vi "Convert Time Stamp to String.vi"(10 "time stamp":timestamp format="%<%Y-%m-%dT%H:%M:%S%8u\nTime zone offset %z>T") -> (3 "date/time string":string)   [LabVIEW 2020, in "infolib.lvlib"]
doc: "Converts time stamp into ISO8601 string."
uses:
  infolib.lvlib
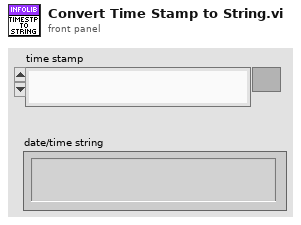
[diagram p1: front panel]
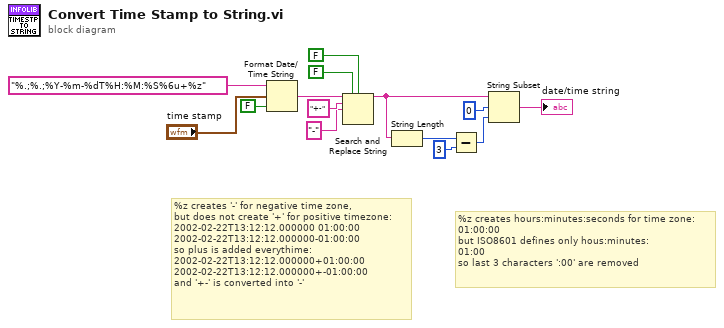
[diagram p0: block diagram]
diagram:
  # "%z creates hours:minutes:seconds for time zone:\n01:00:00\nbut ISO8601 defines only hous:minutes:\n01:00\nso last 3 characters ':00' are removed"
  # "%z creates '-' for negative time zone,\nbut does not create '+' for positive timezone:\n2002-02-22T13:12:12.000000 01:00:00\n2002-02-22T13:12:12.000000-01:00:00\nso plus is added everythime:\n2002-02-22T13:12:12.000000+01:00:00\n2002-02-22T13:12:12.000000+-01:00:00\nand '+-' is converted into '-'"
  n1 = Format Date/Time String(time format string (%c)="%.;%.;%Y-%m-%dT%H:%M:%S%6u+%z" ("format string"), seconds (now)="time stamp", UTC format=FALSE) -> (date/time string=w7:string)
  n2 = Search and Replace String(replace all?=FALSE ("replace all? (F)"), case sensitive?=FALSE ("ignore case? (F)"), input string=w7, search string="+-", replace string="-" ("replace string (\"\")")) -> (result string=w4:string)  [unwired: 3 in, 3 out]
  n3 = String Length(string=w4) -> (length=w5:i32)
  n4 = Subtract(x=w5, y=3 ("length (rest)")) -> (x-y=w2:i32)
  n5 = String Subset(string=w4, offset (0)=0, length (rest)=w2) -> (substring=→"date/time string":string)
